vi "RT Main.vi"() -> ()   [LabVIEW 2018]
doc: "The myRIO Custom FPGA Project template acquires button data from the onboard button and displays the button value on a Boolean indicator. The SYS.RDY indicator shows the FPGA status."
uses:
  <vilib>/Platform/TimedLoop/XDataNode/timing_clust.ctl
  <vilib>/Platform/TimedLoop/XDataNode/nitl_modes.ctl
  <vilib>/Platform/TimedLoop/XDataNode/wakeup.ctl
  <vilib>/myRIO/Instrument Drivers/Onboard IO/DIO/typedefs/DIO Reference.ctl
  <vilib>/myRIO/Common/Instrument Driver Framework/Utilities/typedefs/myRIO Generic Hardware Reference.ctl
  <vilib>/myRIO/Common/Instrument Driver Framework/Utilities/typedefs/Hardware Version Enum.ctl
  <vilib>/myRIO/Common/Instrument Driver Framework/Utilities/typedefs/myRIO v1.0 Reference.ctl
  <vilib>/myRIO/Common/Instrument Driver Framework/Utilities/typedefs/Generic FPGA Reference.ctl
  <vilib>/myRIO/Common/Instrument Driver Framework/myRIO v1.0/DIO/typedefs/DIO Channels List.ctl
  <vilib>/myRIO/Common/Instrument Driver Framework/myRIO v1.0/DIO/typedefs/DIO Channels Enum.ctl
  <vilib>/userdefined/High Color/nirio_resource_hc.ctl
  <vilib>/myRIO/Instrument Drivers/Onboard IO/AI/typedefs/AI Reference.ctl
  <vilib>/myRIO/Common/Instrument Driver Framework/myRIO v1.0/AI/typedefs/AI Channels List.ctl
  <vilib>/myRIO/Common/Instrument Driver Framework/myRIO v1.0/AI/typedefs/AI Channels Enum.ctl
  <vilib>/myRIO/Common/Instrument Driver Framework/Utilities/typedefs/Analog Scaling Constants List.ctl
  <vilib>/myRIO/Common/Instrument Driver Framework/Utilities/typedefs/Analog Scaling Constants.ctl
  <vilib>/myRIO/Instrument Drivers/Onboard IO/AO/typedefs/AO Reference.ctl
  <vilib>/myRIO/Common/Instrument Driver Framework/myRIO v1.0/AO/typedefs/AO Channels List.ctl
  <vilib>/myRIO/Common/Instrument Driver Framework/myRIO v1.0/AO/typedefs/AO Channels Enum.ctl
  <vilib>/myRIO/Common/Instrument Driver Framework/Utilities/vis/Is FPGA Ref Available.vi
  <vilib>/myRIO/Common/Instrument Driver Framework/myRIO v1.0/AI/vis/myRIO v1.1 Open AI.vi
  <vilib>/myRIO/Instrument Drivers/Onboard IO/AI/vis/Read.vi
  <vilib>/myRIO/Common/Instrument Driver Framework/myRIO v1.0/DIO/vis/myRIO v1.1 Open DIO.vi
  <vilib>/myRIO/Instrument Drivers/Onboard IO/DIO/vis/Read.vi
  <vilib>/myRIO/Instrument Drivers/Onboard IO/DIO/vis/Write.vi
  <vilib>/myRIO/Common/Instrument Driver Framework/myRIO v1.0/AO/vis/myRIO v1.1 Open AO.vi
  <vilib>/myRIO/Instrument Drivers/Onboard IO/AO/vis/Write.vi
  <vilib>/myRIO/Common/Instrument Driver Framework/Utilities/vis/Validate Channels.vi
  <vilib>/myRIO/Common/Instrument Driver Framework/myRIO v1.0/AI/vis/myRIO v1.0 Reserve AI.vi
  <vilib>/myRIO/Common/Instrument Driver Framework/myRIO v1.0/DIO/vis/myRIO v1.0 Reserve DIO.vi
  <vilib>/myRIO/Common/Instrument Driver Framework/myRIO v1.0/AO/vis/myRIO v1.0 Reserve AO.vi
  <vilib>/myRIO/Common/Instrument Driver Framework/myRIO v1.0/AI/vis/myRIO v1.0 Build MUX Configuration AI.vi
  <vilib>/myRIO/Common/Instrument Driver Framework/myRIO v1.0/Resource Manager/vis/myRIO v1.0 Reserve Channel List.vi
  <vilib>/myRIO/Common/Instrument Driver Framework/myRIO v1.0/DIO/vis/myRIO v1.0 Build MUX Configuration DIO.vi
  <vilib>/myRIO/Common/Instrument Driver Framework/myRIO v1.0/AO/vis/myRIO v1.0 Build MUX Configuration AO.vi
  <vilib>/myRIO/Common/Instrument Driver Framework/myRIO v1.0/Resource Manager/vis/myRIO v1.0 Reserve Channel.vi
  <vilib>/myRIO/Common/Instrument Driver Framework/myRIO v1.0/Resource Manager/vis/myRIO v1.0 Unreserve Channel.vi
  <vilib>/myRIO/Common/Instrument Driver Framework/myRIO v1.0/Resource Manager/vis/myRIO v1.0 Create Configuration List.vi
  <vilib>/myRIO/Common/Instrument Driver Framework/myRIO v1.0/Resource Manager/vis/myRIO v1.0 Build Mutex Name.vi
  <vilib>/Utility/VariantDataType/GetNumericInfo.vi
  <vilib>/Utility/error.llb/Error Cluster From Error Code.vi
  <vilib>/myRIO/Common/Instrument Driver Framework/myRIO v1.0/myRIO v1.1 Open.vi
  <vilib>/myRIO/Common/Instrument Driver Framework/myRIO v1.0/AI/vis/myRIO v1.0 Get Scaling Constants AI.vi
  <vilib>/myRIO/Common/Instrument Driver Framework/Utilities/vis/IO Manager.vi
  <vilib>/myRIO/Common/Instrument Driver Framework/Utilities/vis/Configuration Manager.vi
  <vilib>/myRIO/Common/Instrument Driver Framework/myRIO v1.0/myRIO v1.0 Close.vi
  <vilib>/myRIO/Common/Instrument Driver Framework/myRIO v1.0/AI/vis/myRIO v1.0 Read AI.vi
  <vilib>/functionblocks/Bistables/SR Bistable/SR Bistable.vi
  <vilib>/myRIO/Common/Instrument Driver Framework/myRIO v1.0/Resource Manager/vis/myRIO v1.0 Configure IO.vi
  <vilib>/myRIO/Common/Instrument Driver Framework/myRIO v1.0/DIO/vis/myRIO v1.0 Write DIO.vi
  <vilib>/myRIO/Common/Instrument Driver Framework/myRIO v1.0/AO/vis/myRIO v1.0 Get Scaling Constants AO.vi
  <vilib>/myRIO/Common/Instrument Driver Framework/myRIO v1.0/AO/vis/myRIO v1.0 Write AO.vi
  <vilib>/Utility/file.llb/Write Delimited Spreadsheet (string).vi
  <vilib>/functionblocks/Counter/Pulse Timer/Pulse Timer.vi
  <vilib>/myRIO/Common/Instrument Driver Framework/myRIO v1.0/DIO/vis/myRIO v1.0 Read DIO.vi
  <vilib>/Platform/TimedLoop/XDataNode/XDataNode.xnode
  <vilib>/myRIO/Express VI/Onboard IO/AI/AI Express VI.xnode
  <vilib>/myRIO/Instrument Drivers/Onboard IO/AI/vis/myRIO AI Open.xnode
  <vilib>/functionblocks/FB Core/FB Core.xnode
  <vilib>/myRIO/Express VI/Onboard Devices/LED/LED Express VI.xnode
  <vilib>/myRIO/Instrument Drivers/Onboard IO/DIO/vis/myRIO DIO Open.xnode
  <vilib>/myRIO/Express VI/Onboard IO/AO/AO Express VI.xnode
  <vilib>/myRIO/Instrument Drivers/Onboard IO/AO/vis/myRIO AO Open.xnode
  <vilib>/myRIO/Express VI/Onboard IO/DO/DO Express VI.xnode
  <vilib>/myRIO/Express VI/Onboard IO/DI/DI Express VI.xnode
  <vilib>/myRIO/Instrument Drivers/Onboard IO/AI/AI.lvlib
  <vilib>/myRIO/Instrument Drivers/Onboard IO/AO/AO.lvlib
  <vilib>/myRIO/Instrument Drivers/Onboard IO/DIO/DIO.lvlib
  <vilib>/Platform/TimedLoop/XDataNode/XDNodeRunTimeDep.lvlib
  <vilib>/functionblocks/NI_FunctionBlock Libraries.lvlib
panel:
  out "Pump out":bool
  in  "Pump Test":bool
  out "Bamocar Temp Threshold":bool
  out "RTD Status LED":bool
  out "RFE Indicator":bool
  out "AIR + Boolean":bool
  out "AIR +(A9)":dbl
  out "RTD Button":bool
  out "RTD Brake":bool
  out "EN Indicator":bool
  out "RTD Buzzer":bool
  in  "Buzzer test":bool
  in  "RTD Brake Test":bool
  in  "RFE  Test":bool
  in  "EN Test":bool
  out "APPS1 (V) Input (B/AI0 (Pin 3))":dbl
  out "APPS2 Scaled Up (V)":dbl
  out "APPS1 Scaled Up (V)":dbl
  out "APPS2 (V) Input (B/AI1 (Pin 5))":dbl
  out "APPS fault":bool
  out "APPS2 %":dbl
  out "APPS1 %":dbl
  out "APPS Output (V)":dbl
  out "APPS output %":dbl
  out "Accelaration":dbl(knob) scale=0.0..100.0
  out "APPS1":dbl(knob) scale=0.0..100.0
  out "APPS2":dbl(knob) scale=0.0..100.0
  out "APPS pedal travel %":dbl
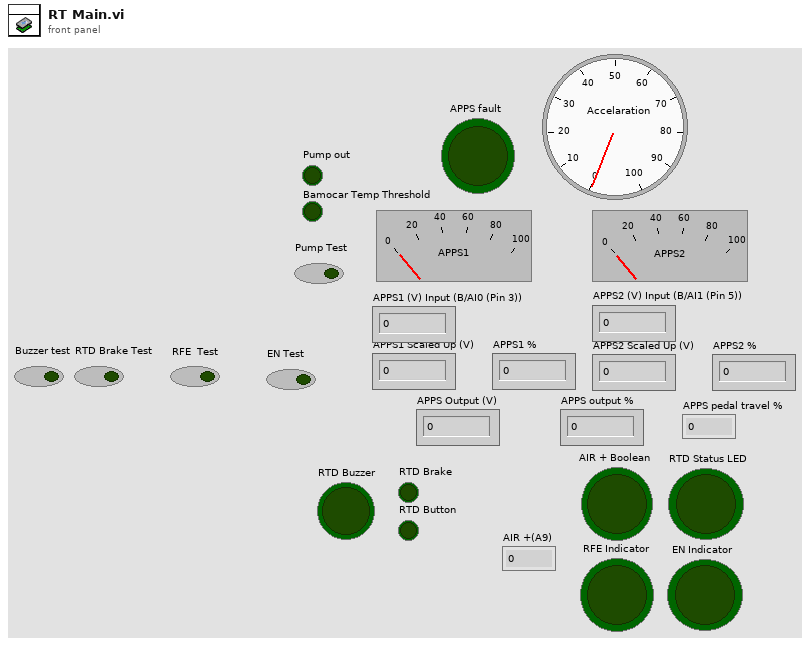
[diagram p1: front panel]
types:
  T1 = typedef "XDNodeRunTimeDep.lvlib/timing_clust.ctl" = cluster{"Expected End [f-1]":u64, "Actual End [f-1]":u64, "Finished Late? [f-1]":bool, "Expected End [i-1]":u64, "Actual End [i-1]":u64, "Finished Late? [i-1]":bool, "Expected Start [i]":u64, "Actual Start [i]":u64, "Expected Start [f]":u64, "Actual Start [f]":u64, "Source Name":string, "Structure Name":string, "Period":i64, "Deadline":i64, "Offset":i64, "Start":i64, "Priority":i32, "Timeout":i32, "Mode":T2, "Wakeup Reason":T3, "Error":errorcluster, "Source Type":string, "Secondary Source Type":string, "Global End Time":u64, "Global Start Time":u64, "Frame Duration":u64, "Iteration Duration":u64, "Assigned CPU":i32, "I/O Scan Engine Mode":u32}
  T2 = typedef "XDNodeRunTimeDep.lvlib/nitl_modes.ctl" = enum32{"No Change", "Process missed periods, maintain original phase", "Discard missed periods, maintain original phase", "Process missed periods, ignore original phase", "Discard missed periods, ignore original phase"}
  T3 = typedef "XDNodeRunTimeDep.lvlib/wakeup.ctl" = enum32{"Normal", "Aborted", "Asynchronous wakeup", "Timing source error", "Timed loop error", "Timeout"}
  T4 = typedef "AI.lvlib/AI Reference.ctl" = cluster{"myRIO Reference":T5, "AI Channels List":T9, "AI Scaling Constants List":T11}
  T5 = typedef "myRIO Generic Hardware Reference.ctl" = cluster{"myRIO Model":T6, "myRIO Hardware Reference":T7}
  T6 = typedef "Hardware Version Enum.ctl" = enum16{"Unknown", "myRIO-1900", "myRIO-1950", "roboRIO", "NI ELVIS RIO CM", "ELVIS III"}
  T7 = typedef "myRIO v1.0 Reference.ctl" = cluster{"Generic FPGA Reference":T8, "Allow multiple opens":bool}
  T8 = typedef "Generic FPGA Reference.ctl" = refnum<k20>
  T9 = typedef "AI Channels List.ctl" = T10[]
  T10 = typedef "AI Channels Enum.ctl" = enum16{"Not Connected", "AudioIn/Left", "AudioIn/Right", "C/AI0", "C/AI1", "A/AI0", "A/AI1", "A/AI2", "A/AI3", "A/AI4", "A/AI5", "A/AI6", "A/AI7", "B/AI0", "B/AI1", "B/AI2", "B/AI3", "B/AI4", "B/AI5", "B/AI6", "B/AI7", "AI/AI0", "AI/AI1", "AI/AI2", "AI/AI3", "A/AI0 (DIFF)", "A/AI1 (DIFF)", "A/AI2 (DIFF)", "A/AI3 (DIFF)", "B/AI0 (DIFF)", "B/AI1 (DIFF)", "B/AI2 (DIFF)", "B/AI3 (DIFF)"}
  T11 = typedef "Analog Scaling Constants List.ctl" = T12[]
  T12 = typedef "Analog Scaling Constants.ctl" = cluster{"LSB Weight (Volts)":dbl, "Offset (Volts)":dbl, "Signed?":bool}
  T13 = typedef "nirio_resource_hc.ctl" = tag
  T14 = typedef "DIO.lvlib/DIO Reference.ctl" = cluster{"myRIO Reference":T5, "DIO Channels List":T15}
  T15 = typedef "DIO Channels List.ctl" = T16[]
  T16 = typedef "DIO Channels Enum.ctl" = enum16{"Not Connected", "C/DIO0", "C/DIO1", "C/DIO2", "C/DIO3", "C/DIO4", "C/DIO5", "C/DIO6", "C/DIO7", "A/DIO0", "A/DIO1", "A/DIO2", "A/DIO3", "A/DIO4", "A/DIO5", "A/DIO6", "A/DIO7", "A/DIO8", "A/DIO9", "A/DIO10", "A/DIO11", "A/DIO12", "A/DIO13", "A/DIO14", "A/DIO15", "A/DIO16", "A/DIO17", "A/DIO18", "A/DIO19", "B/DIO0", "B/DIO1", "B/DIO2", "B/DIO3", "B/DIO4", "B/DIO5", "B/DIO6", "B/DIO7", "B/DIO8", "B/DIO9", "B/DIO10", "B/DIO11", "B/DIO12", "B/DIO13", "B/DIO14", "B/DIO15", "B/DIO16", "B/DIO17", "B/DIO18", "B/DIO19", "LED0", "LED1", "LED2", "LED3", "Button0", "DIO/DIO0", "DIO/DIO1", "DIO/DIO2", "DIO/DIO3", "DIO/DIO4", "DIO/DIO5", "DIO/DIO6", "DIO/DIO7", "DIO/DIO8", "DIO/DIO9", "SPI/CS0", "SPI/CS1", "SPI/CS2", "SPI/CS3", "LED RADIO (Green)", "LED RADIO (Red)", "LED COMM (Green)", "LED COMM (Red)", "LED MODE (Green)", "LED MODE (Red)"}
  T17 = typedef "AO.lvlib/AO Reference.ctl" = cluster{"myRIO Reference":T5, "AO Channel List":T18, "AO Scaling Constant List":T11}
  T18 = typedef "AO Channels List.ctl" = T19[]
  T19 = typedef "AO Channels Enum.ctl" = enum16{"Not Connected", "AudioOut/Left", "AudioOut/Right", "C/AO0", "C/AO1", "A/AO0", "A/AO1", "B/AO0", "B/AO1"}
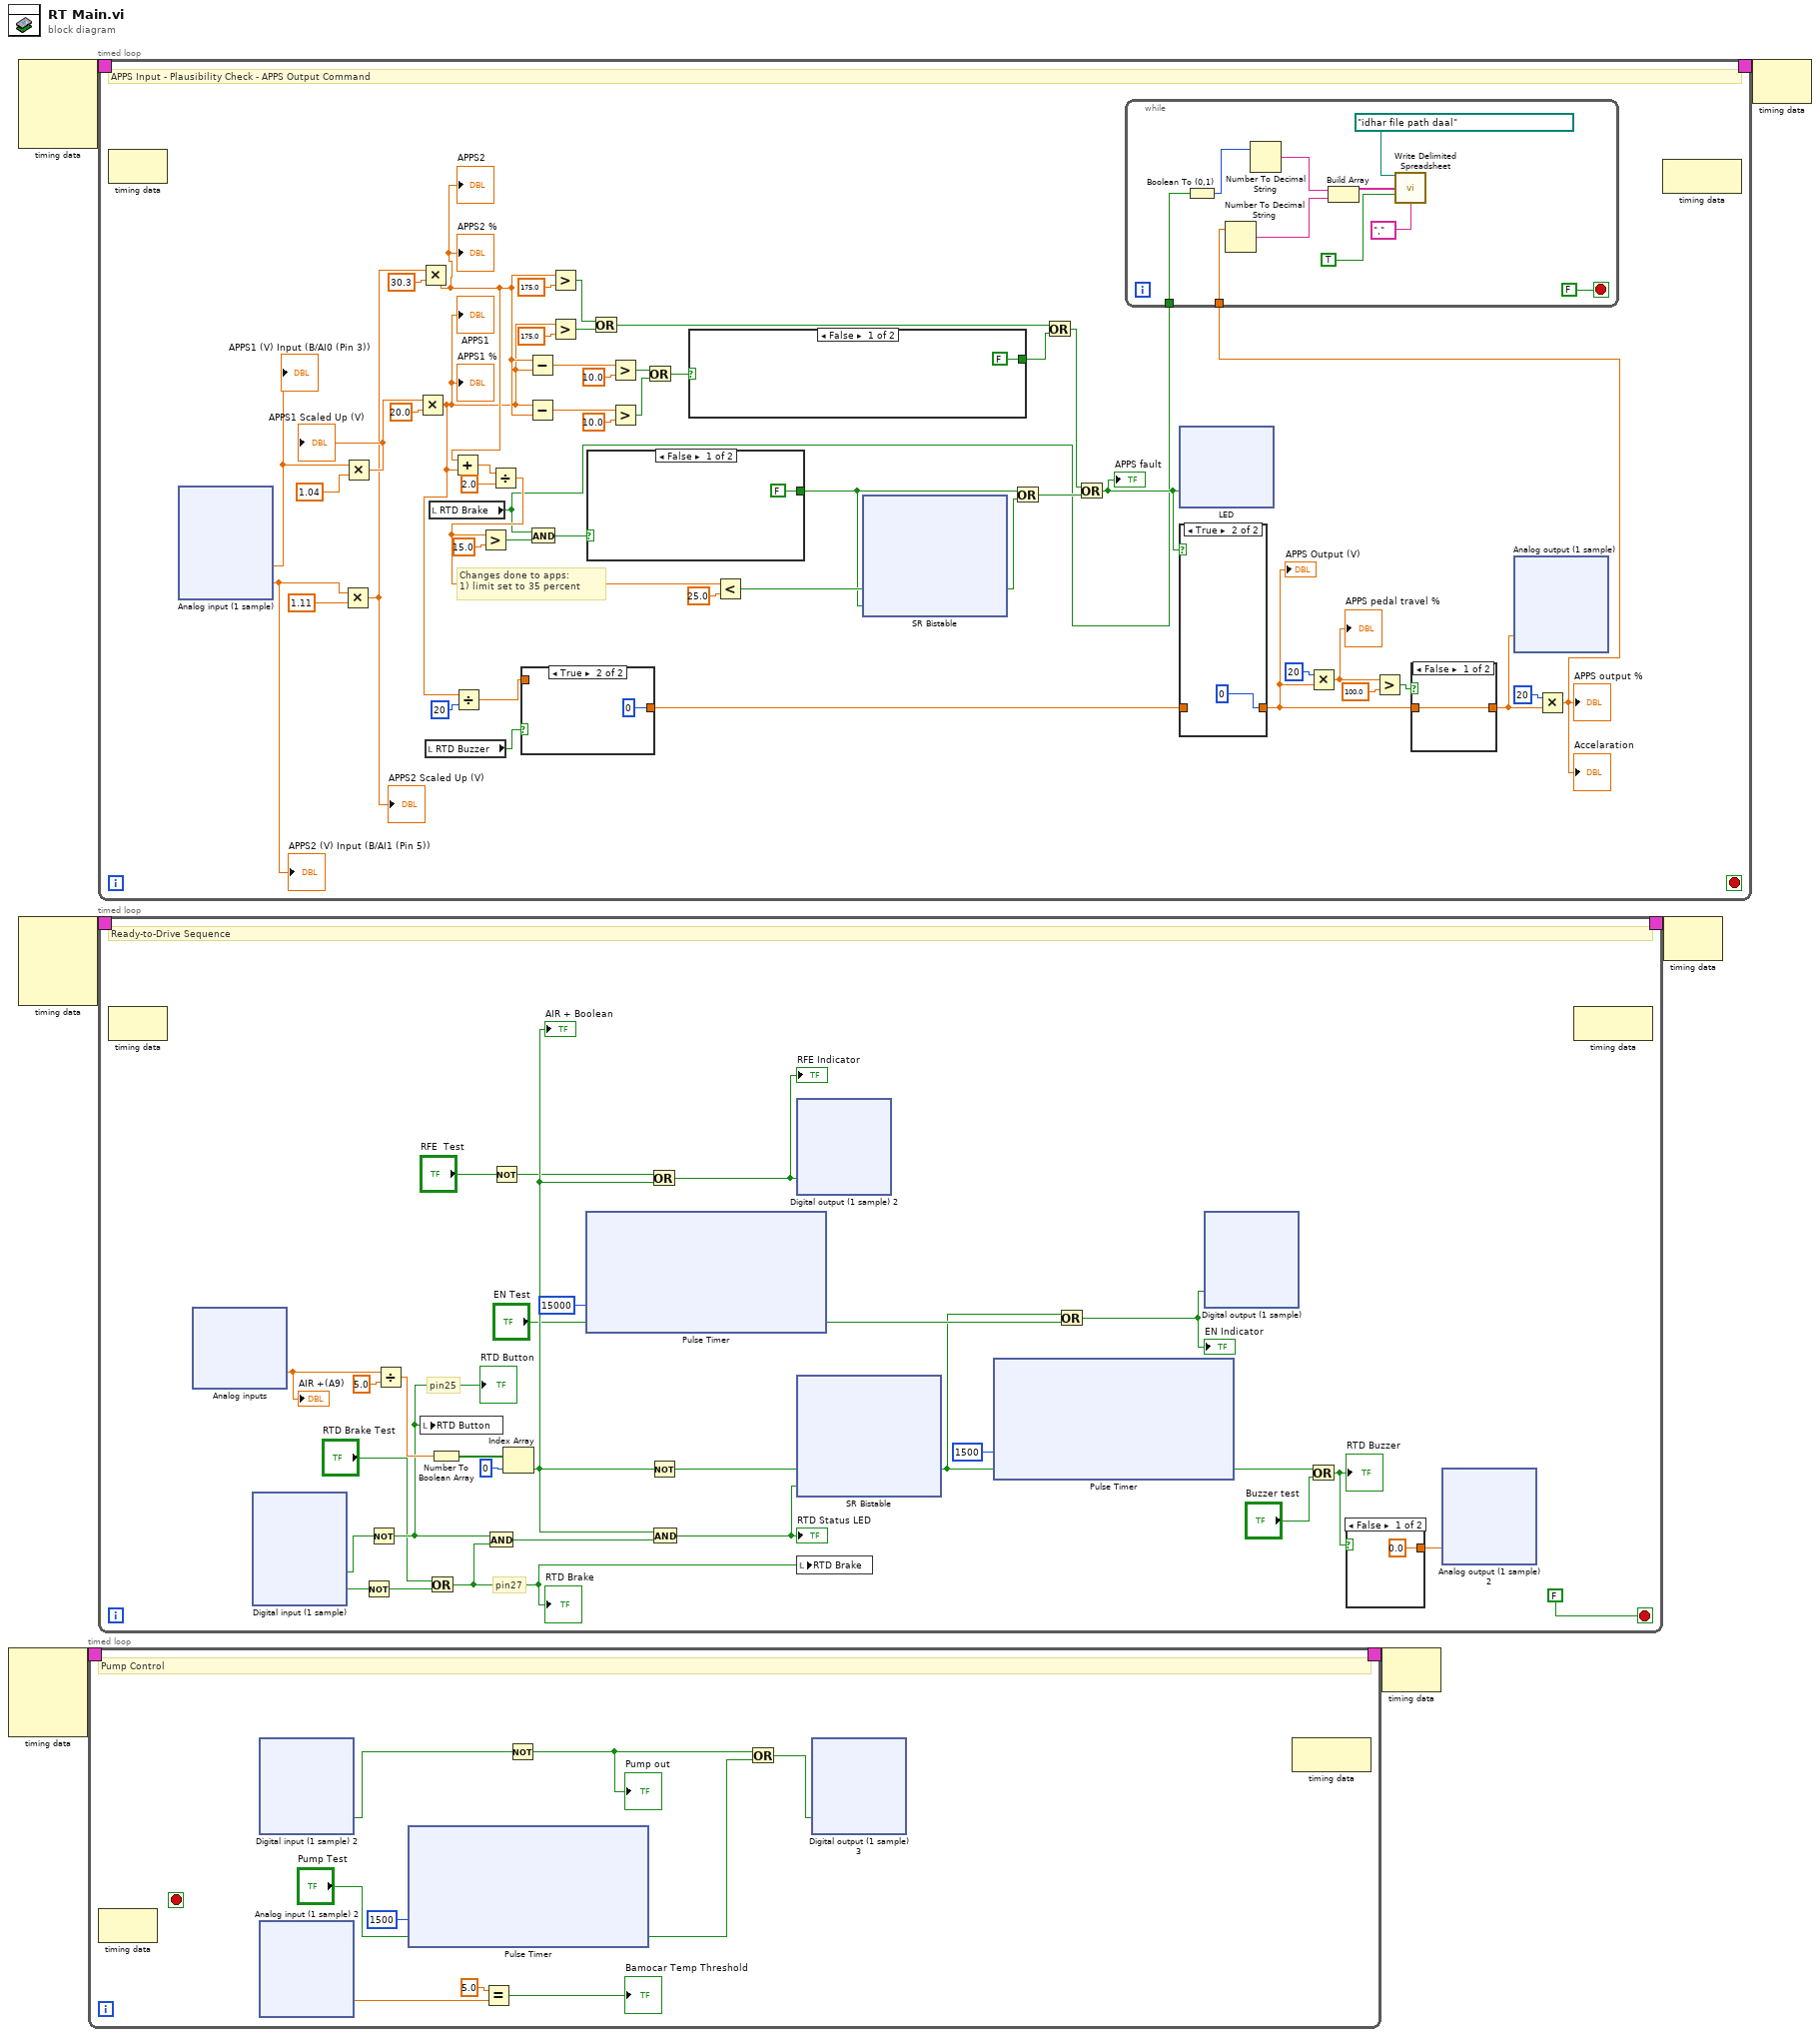
[diagram p0: block diagram]
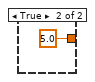
[diagram p2: hidden frame]
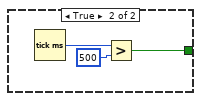
[diagram p3: hidden frame]
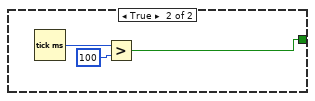
[diagram p4: hidden frame]
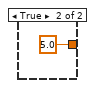
[diagram p6: hidden frame]
diagram:
  n1 = node-c288() -> (w2:T1)  [unwired: 4 in]
  n2 = node-c288() -> (w6:T1)  [unwired: 4 in]
  n3 = node-c288() -> (w4:T1)  [unwired: 4 in]
  n4 = timed-loop {
    timing: w2 -> [_]
    timing-out: [_] -> w1
    stop <- _ stop-if-true
    # "Pump Control"
    n5 = node-c288() -> ()  [unwired: 1 in, 1 out]
    n6 = xnode "Digital input (1 sample) 2"() -> ("B/DIO9 (Pin 29)"=w15:bool)  [unwired: 1 in, 1 out]
    n7 = xnode "Analog input (1 sample) 2"() -> ("Pump Bamocar (A/AI3 (Pin 9))"=w10:dbl)  [unwired: 1 in, 1 out]
    n8 = xnode "Pulse Timer"("preset time (ms)"=1500, "input"="Pump Test") -> ("output"=w12:bool)  [unwired: 1 in, 2 out]
    n9 = Equal?(x=5.0, y=w10) -> (x = y?=→"Bamocar Temp Threshold":bool)
    n10 = Not(x=w15) -> (.not. x?=w7:bool)
    "Pump out" <- w7
    n11 = Or(x=w7, y=w12) -> (x .or. y?=w11:bool)
    n12 = xnode "Digital output (1 sample) 3"("Pump out (B/DIO8 (Pin 27))"=w11) -> ()  [unwired: 1 in, 1 out]
    n13 = node-c288() -> ()  [unwired: 1 in, 1 out]
  }
  n14 = timed-loop {
    timing: w6 -> [_]
    timing-out: [_] -> w5
    stop <- _ stop-if-true
    # "Changes done to apps:\n1) limit set to 35 percent"
    # "APPS Input - Plausibility Check - APPS Output Command"
    n15 = node-c288() -> ()  [unwired: 1 in, 1 out]
    n16 = xnode "Analog input (1 sample)"() -> ("APPS 1 Input (B/AI0 (Pin 3))"=w197:dbl, "APPS 2 Input (B/AI1 (Pin 5))"=w196:dbl)  [unwired: 1 in, 1 out]
    "APPS1 (V) Input (B/AI0 (Pin 3))" <- w197
    "APPS2 (V) Input (B/AI1 (Pin 5))" <- w196
    n17 = Multiply(x=w196, y=1.11) -> (x*y=w173:dbl)
    "APPS2 Scaled Up (V)" <- w173
    n18 = Multiply(x=w197, y=1.04) -> (x*y=w174:dbl)
    "APPS1 Scaled Up (V)" <- w174
    n19 = Multiply(x=w174, y=20.0) -> (x*y=w171:dbl)
    "APPS1 %" <- w171
    "APPS1" <- w171
    n20 = Multiply(x=w173, y=30.3) -> (x*y=w172:dbl)
    "APPS2 %" <- w172
    "APPS2" <- w172
    n21 = local read "RTD Buzzer"() -> (w193:bool)
    n22 = local read "RTD Brake"() -> (w167:bool)
    n23 = Add(x=w172, y=w171) -> (x+y=w177:dbl)
    n24 = Divide(x=w171, y=20) -> (x/y=w170:dbl)
    n25 = Divide(x=w177, y=2.0) -> (x/y=w175:dbl)
    n26 = Greater?(x=w175, y=15.0) -> (0:w199:bool)
    n27 = case shown="True" w193 {
      tunnel: [w278 0] -> w192
      tunnel: w170 -> [w278 _]
      frame False {
      }
      frame True {
      }
    }
    n28 = Subtract(x=w172, y=w171) -> (x-y=w213:dbl)
    n29 = Subtract(x=w171, y=w172) -> (x-y=w201:dbl)
    n30 = And(x=w167, y=w199) -> (x .and. y?=w180:bool)
    n31 = Greater?(x=w172, y=175.0) -> (0:w210:bool)
    n32 = Greater?(x=w171, y=175.0) -> (0:w209:bool)
    n33 = case shown="False" w180 {
      tunnel: [FALSE w229] -> w179
      frame False {
      }
      frame True {
        n34 = Tick Count (ms)() -> (millisecond timer value=w231:u32)
        n35 = Greater?(x=w231, y=u32 500) -> (0:w229:bool)
      }
    }
    n36 = Or(x=w210, y=w209) -> (x .or. y?=w208:bool)
    n37 = Greater?(x=w213, y=10.0) -> (0:w214:bool)
    n38 = Greater?(x=w201, y=10.0) -> (0:w202:bool)
    n39 = Or(x=w214, y=w202) -> (x .or. y?=w187:bool)
    n40 = case shown="False" w187 {
      tunnel: [FALSE w275] -> w186
      frame False {
      }
      frame True {
        n41 = Tick Count (ms)() -> (millisecond timer value=w277:u32)
        n42 = Greater?(x=w277, y=u32 100) -> (0:w275:bool)
      }
    }
    n43 = Less?(x=w175, y=25.0) -> (x < y?=w184:bool)
    n44 = xnode "SR Bistable"("reset"=w184, "set"=w179) -> ("output"=w185:bool)  [unwired: 1 in, 1 out]
    n45 = Or(x=w179, y=w185) -> (x .or. y?=w182:bool)
    n46 = Or(x=w208, y=w186) -> (x .or. y?=w183:bool)
    n47 = Or(x=w183, y=w182) -> (x .or. y?=w181:bool)
    "APPS fault" <- w181
    n48 = xnode "LED"("LED0"=w181) -> ()  [unwired: 1 in, 1 out]
    n49 = case shown="True" w181 {
      tunnel: w192 -> [w282 _]
      tunnel: [w282 0] -> w191
      frame False {
      }
      frame True {
      }
    }
    "APPS Output (V)" <- w191
    n50 = Multiply(x=20, y=w191) -> (x*y=w178:dbl)
    "APPS pedal travel %" <- w178
    n51 = Greater?(x=w178, y=100.0) -> (0:w194:bool)
    n52 = case shown="False" w194 {
      tunnel: [w280 5.0 ("APPS output %")] -> w189
      tunnel: w191 -> [w280 _]
      frame False {
      }
      frame True {
      }
    }
    n53 = xnode "Analog output (1 sample)"("APPS Output (B/AO0 (Pin 2))"=w189) -> ()  [unwired: 1 in, 1 out]
    n54 = Multiply(x=20, y=w189) -> (x*y=w168:dbl)
    "APPS output %" <- w168
    "Accelaration" <- w168
    n55 = while {
      tunnel: w168 -> [w224]
      tunnel: w167 -> [w223]
      stop <- FALSE stop-if-true
      n56 = Boolean To (0,1)(Boolean=w223) -> (0, 1=w222:i16)
      n57 = Number To Decimal String(number=w224) -> (decimal integer string=w225:string)  [unwired: 1 in]
      n58 = Number To Decimal String(number=w222) -> (decimal integer string=w221:string)  [unwired: 1 in]
      n59 = Build Array(w221, w225) -> (w220:string[])
      n60 = call-poly <vilib>:"Write Delimited Spreadsheet.vi"("file path (dialog if empty)"=path "idhar file path daal", "1D data"=w220, "append to file? (new file:F)"=TRUE, "delimiter (\\t)"="," ("delimiter (\\t)")) -> ()  [unwired: 10 in, 2 out]
    }
    n61 = node-c288() -> ()  [unwired: 1 in, 1 out]
  }
  n62 = timed-loop {
    timing: w4 -> [_]
    timing-out: [_] -> w3
    stop <- FALSE stop-if-true
    # "pin27"
    # "pin25"
    # "Ready-to-Drive Sequence"
    n63 = node-c288() -> ()  [unwired: 1 in, 1 out]
    n64 = xnode "Analog inputs"() -> ("AIR + (B/AI2 (Pin 7))"=w417:dbl)  [unwired: 1 in, 1 out]
    "AIR +(A9)" <- w417
    n65 = xnode "Digital input (1 sample)"() -> ("RTD Button (B/DIO2 (Pin 15))"=w416:bool, "RTD Brake (B/DIO3 (Pin 17))"=w415:bool)  [unwired: 1 in, 1 out]
    n66 = Not(x=w415) -> (.not. x?=w409:bool)
    n67 = Not(x=w416) -> (.not. x?=w413:bool)
    "RTD Button" <- w413
    n68 = Divide(x=w417, y=5.0) -> (x/y=w421:dbl)
    n69 = local write "RTD Button"(w413) -> ()
    n70 = Or(x="RTD Brake Test", y=w409) -> (x .or. y?=w408:bool)
    "RTD Brake" <- w408
    n71 = Number To Boolean Array(number=w421) -> (Boolean array=w422:bool[])
    n72 = And(x=w413, y=w408) -> (x .and. y?=w418:bool)
    n73 = Not(x="RFE  Test") -> (.not. x?=w395:bool)
    n74 = Index Array(array=w422, index=0) -> (element=w407:bool)
    "AIR + Boolean" <- w407
    n75 = xnode "Pulse Timer"("preset time (ms)"=15000, "input"="EN Test") -> ("output"=w403:bool)  [unwired: 1 in, 2 out]
    n76 = Or(x=w395, y=w407) -> (x .or. y?=w406:bool)
    "RFE Indicator" <- w406
    n77 = Not(x=w407) -> (.not. x?=w411:bool)
    n78 = And(x=w407, y=w418) -> (x .and. y?=w412:bool)
    "RTD Status LED" <- w412
    n79 = xnode "Digital output (1 sample) 2"("RFE (B/DIO0 (Pin 11))"=w406) -> ()  [unwired: 1 in, 1 out]
    n80 = xnode "SR Bistable"("reset"=w411, "set"=w412) -> ("output"=w400:bool)  [unwired: 1 in, 1 out]
    n81 = local write "RTD Brake"(w408) -> ()
    n82 = xnode "Pulse Timer"("preset time (ms)"=1500, "input"=w400) -> ("output"=w398:bool)  [unwired: 1 in, 2 out]
    n83 = Or(x=w400, y=w403) -> (x .or. y?=w402:bool)
    "EN Indicator" <- w402
    n84 = xnode "Digital output (1 sample)"("EN (B/DIO1 (Pin 13))"=w402) -> ()  [unwired: 1 in, 1 out]
    n85 = Or(x=w398, y="Buzzer test") -> (x .or. y?=w397:bool)
    "RTD Buzzer" <- w397
    n86 = case shown="False" w397 {
      tunnel: [0.0 ("y") 5.0 ("y")] -> w414
      frame False {
      }
      frame True {
      }
    }
    n87 = xnode "Analog output (1 sample) 2"("RTD - Buzzer (B/AO1 (Pin 4))"=w414) -> ()  [unwired: 1 in, 1 out]
    n88 = node-c288() -> ()  [unwired: 1 in, 1 out]
  }
  n89 = node-c288(w1) -> ()  [unwired: 1 out]
  n90 = node-c288(w3) -> ()  [unwired: 1 out]
  n91 = node-c288(w5) -> ()  [unwired: 1 out]
